vi "Controller_PP.vi"(0 "Zdot":dbl=1.0, 1 "Z":dbl=1.0, 5 "State-Space Model":T1 {"Transport Delay" format="%.2f"; "D" format="%#.2g"; "C" format="%#.2g"; "B" format="%#.2g"; "A" format="%#.2g"; "properties"."Sampling Time" format="%#.6p"; "properties"."Output Delays" format="%.4f"; "properties"."Input Delays" format="%.4f"}, 7 "Real":dbl(knob)=-3.4076115316471642 scale=0.0..-22.0 scale format="%#_4g", 9 "Imaginary":dbl(knob)=-10.013861291935129 scale=0.0..-20.0 scale format="%#_4g", 12 "state x(k)":dbl[](array[numeric])) -> (2 "Setpoints":dbl[](array[numeric]), 3 "u(k)":dbl format="%.2f", 4 "X * Y":dbl, 6 "Closed-Loop Step Response":cluster{"time":dbl[], dbl[]}[](graph), 8 "State Trajectory Graph":cluster{"time":dbl[], dbl[]}[](graph), 10 "Gain":dbl[](array[numeric]), 13 "Desired Poles":cdb[](array[numeric])=[-4.951252167649562+0.0i, -3.4076115316471642-10.013861291935129i, -3.4076115316471642+10.013861291935129i] format="%.2f", 14 "Actual Poles":cdb[](array[numeric])=[-4.9512521676495505+0.0i, -3.4076115316471447-10.013861291935113i, -3.4076115316471447+10.013861291935113i] format="%.2f")   [LabVIEW 2011]
uses:
  <vilib>/addons/Control Design/_Model Construction/Model Typedefs.llb/CD State Space Model (MIMO).ctl
  <vilib>/addons/Control Design/_Model Construction/Model Typedefs.llb/CD General Elements.ctl
  <vilib>/Simulation/Implementation/Shared/SIMSCR Execution Mode.ctl
  <vilib>/Simulation/Scripting/Companion Diagram/SimConfigNode/SimParams.ctl
  <vilib>/Simulation/Scripting/Companion Diagram/SimConfigNode/_simSolvers.ctl
  <vilib>/Simulation/Param Hierarchy/Typedefs/SIMPH Param Control Actions.ctl
  <vilib>/Simulation/Implementation/Shared/NILVSim_Manager.vi
  <vilib>/Simulation/Implementation/Shared/NILVSim_ParamChanged.vi
  <vilib>/Simulation/Implementation/Shared/NILVSim_FinalizeModel.vi
  <vilib>/Simulation/Implementation/Shared/SIM Unbundle Sim Info.vi
  <vilib>/Simulation/Implementation/Shared/NILVSim_GetModelError.vi
  <vilib>/Simulation/Implementation/Shared/SIM SimErrorHandler.vi
  <vilib>/Simulation/Implementation/Shared/SIM Bundle Sim Info.vi
  <vilib>/Simulation/Implementation/Shared/NILVSim_Initialize.vi
  <vilib>/Analysis/baseanly.llb/Real Dot Product.vi
  <vilib>/Simulation/Scripting/Companion Diagram/SimConfigNode/SimDog.xnode
  <vilib>/Analysis/NI_AALBase.lvlib
  <vilib>/Simulation/Implementation/Shared/NI_SIM_Implementation.lvlib
  <vilib>/addons/Control Design/_Model Construction/NI_LinSys_Model Typedefs.lvlib
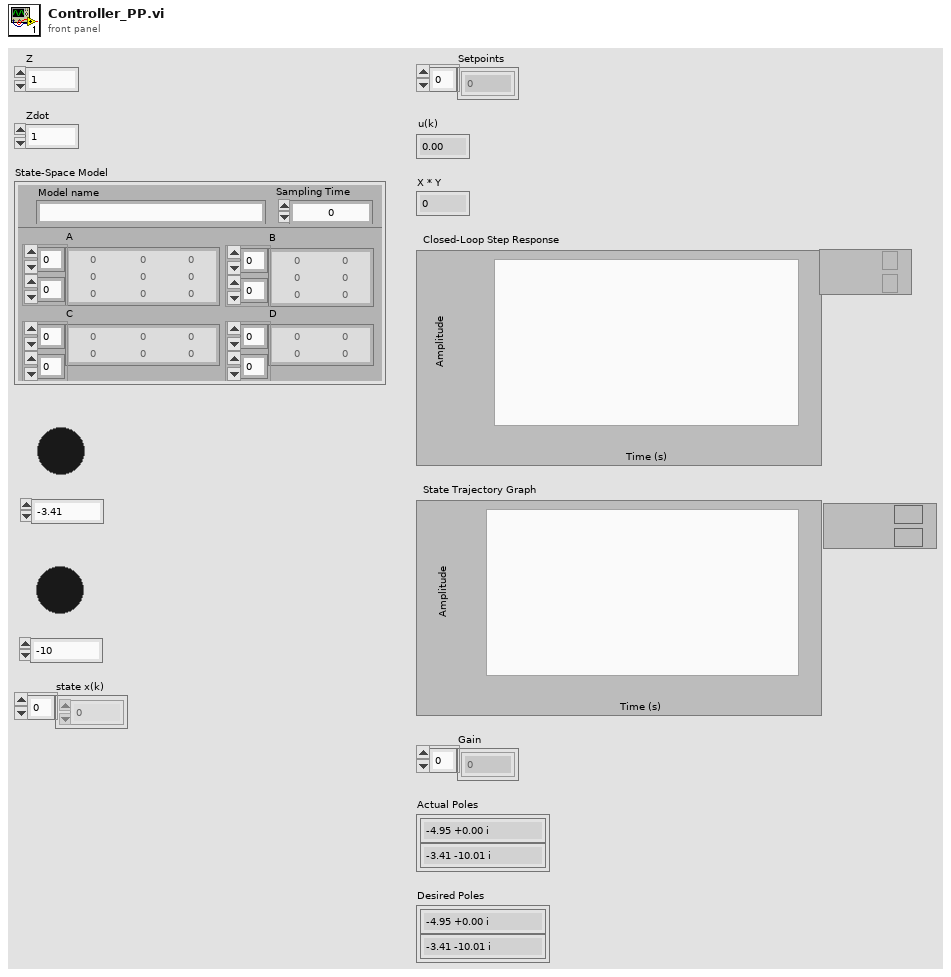
[diagram p1: front panel]
types:
  T1 = typedef "NI_LinSys_Model Typedefs.lvlib/CD State Space Model (MIMO).ctl" = cluster{"properties":T2, "A":dbl[][], "B":dbl[][], "C":dbl[][], "D":dbl[][], "StateNames":string[], "Transport Delay":dbl[][]}
  T2 = typedef "NI_LinSys_Model Typedefs.lvlib/CD General Elements.ctl" = cluster{"Model name":string, "Input names":string[], "Output names":string[], "Input Delays":dbl[], "Output Delays":dbl[], "Sampling Time":dbl, "Notes":string}
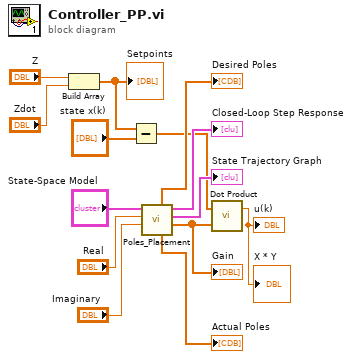
[diagram p0: block diagram]
diagram:
  n1 = Build Array("Z", "Zdot") -> (w6:dbl[])
  "Setpoints" <- w6
  n2 = Subtract ("Subtract.vi")(x=w6, y="state x(k)") -> (x-y=w7:dbl[])
  n3 = call "Poles_Placement.vi"("Imaginary"="Imaginary", "Real"="Real", "State-Space Model"="State-Space Model") -> ("Gain"=w14:dbl[], "State Trajectory Graph"=→"State Trajectory Graph":cluster{"time":dbl[], dbl[]}[], "Closed-Loop Step Response"=→"Closed-Loop Step Response":cluster{"time":dbl[], dbl[]}[], "Actual Poles"=→"Actual Poles":cdb[], "Desired Poles"=→"Desired Poles":cdb[])  [unwired: 4 in]
  "Gain" <- w14
  n4 = call-poly <vilib>:"Dot Product.vi"("Y Vector"=w14, "X Vector"=w7) -> ("X * Y"=→"u(k)" →"X * Y":dbl)  [unwired: 1 out]
